vi "SubPanelVI2.vi"(8 "error in (no error)":errorcluster, 11 "UI in":refnum<class "UI.lvclass">) -> (0 "error out":errorcluster, 3 "UI out":refnum<class "UI.lvclass">)   [LabVIEW 2018]
uses:
  UI/UI.lvclass
  UI/UI.lvclass/UI.ctl
  UI/getUIData.vi
  UI/setEmbeddedVI.vi
panel:
  out "Waveform Chart":dbl(graph)
  in  "Stop Button":bool
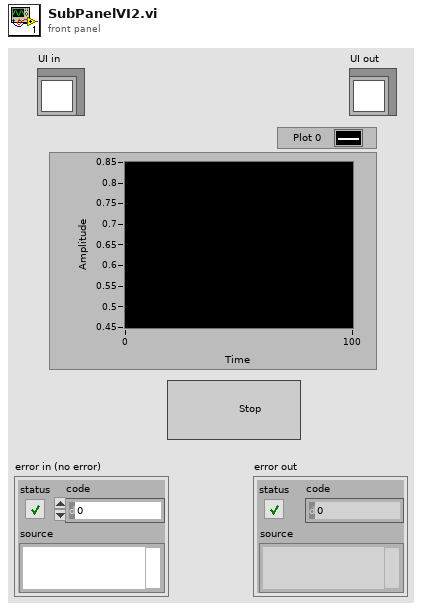
[diagram p1: front panel]
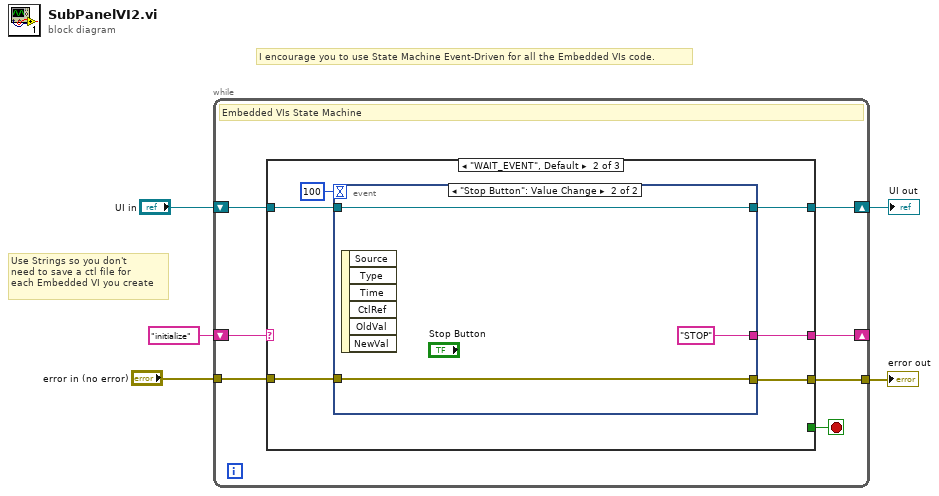
[diagram p0: block diagram]
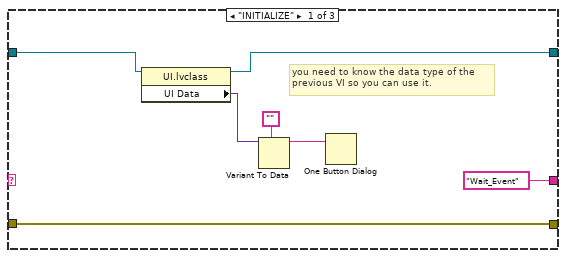
[diagram p2: hidden frame]
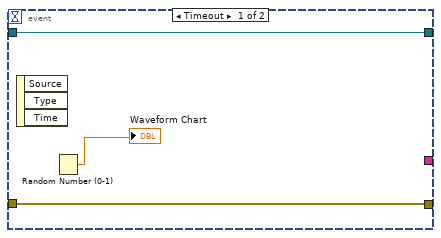
[diagram p3: hidden frame]
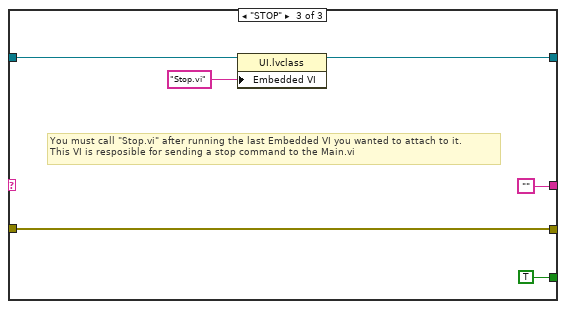
[diagram p4: hidden frame]
diagram:
  # "I encourage you to use State Machine Event-Driven for all the Embedded VIs code."
  # "Use Strings so you don't\nneed to save a ctl file for\neach Embedded VI you create"
  n1 = while {
    shift-right: [w11] -> w5
    shift-left: "UI in" -> [w12]
    tunnel: [w10] -> w3
    tunnel: "error in (no error)" -> [w9]
    shift-right: [w7] -> _
    shift-left: "initialize" -> [w8]
    stop <- w6 stop-if-true
    # "Embedded VIs State Machine"
    n2 = case shown="\"WAIT_EVENT\", Default" w8 {
      tunnel: w12 -> [w15 w25 w37]
      tunnel: [w14 w24 w33] -> w11
      tunnel: [w19 w23 w36] -> w10
      tunnel: w9 -> [w19 w22 w36]
      tunnel: ["Wait_Event" w20 ""] -> w7
      tunnel: [_ _ TRUE] -> w6
      frame "INITIALIZE" {
        # "you need to know the data type of the\nprevious VI so you can use it."
        n3 = property class="UI.lvclass"(reference=w15) -> (reference out=w14:refnum<class "UI.lvclass">, "UI Data"=w18:variant)  [unwired: 1 in, 1 out]
        n4 = Variant To Data(type="", Variant=w18) -> (data=w16:string)  [unwired: 1 in, 1 out]
        n5 = One Button Dialog(message=w16) -> ()  [unwired: 1 in, 1 out]
      }
      frame "WAIT_EVENT", Default {
        n6 = event shown="[1] \"Stop Button\": Value Change" {
          selector: _ -> [_ _]
          dyn-events: _ -> [_ _]
          timeout: 100 -> [_ _]
          tunnel: [w28 w31] -> w24
          tunnel: w25 -> [w28 w31]
          tunnel: [w27 w30] -> w23
          tunnel: w22 -> [w27 w30]
          tunnel: [_ "STOP"] -> w20
          event Timeout {
            n7 = event-data() -> ()  [unwired: 1 in, 3 out]
            n8 = Random Number (0-1)() -> (number: 0 to 1=→"Waveform Chart":dbl)
          }
          event "Stop Button": Value Change {
            n9 = event-data() -> ()  [unwired: 1 in, 6 out]
          }
        }
      }
      frame "STOP" {
        # "You must call \"Stop.vi\" after running the last Embedded VI you wanted to attach to it.\nThis VI is resposible for sending a stop command to the Main.vi"
        n10 = property class="UI.lvclass"(reference=w37, "Embedded VI"="Stop.vi" ("String <Replace Me>")) -> (reference out=w33:refnum<class "UI.lvclass">)  [unwired: 1 in, 1 out]
      }
    }
  }
  "UI out" <- w5
  "error out" <- w3
